vi "decode-from-json.vi"(8 "sensor-options-json":string, 9 "serial-port-json":string, 10 "data-logging-json":string, 11 "filepath-json":string) -> (0 "Sensor Option Recall":T1={"Display Units"="log", "Zero Offset"=2.62, "Sensor Min"=0.0, "Sensor Max"=500.0, "Signal Min"=0.0, "Signal Max"=100.0, "Conversion Factor"=0.0}, 1 "Serial Port Recall":T2={"COM Port (COM10)"="COM10", "baud rate (19200)"=19200, "Simulate Hardware"=FALSE} {"baud rate (19200)" max=115200 step=1200}, 2 "Datalogging Recall":T3={"data-precision"=3, "Include Date"=FALSE, "Include Timestamp"=TRUE, "Include Milliseconds"=FALSE, "sample-rate (Hz)"=4.0, "Logging Active"=TRUE}, 3 "Filepath Recall":T4={"Log Filepath Source"=enum."Application Relative (Auto)", "Log File Path (Manual)"=path "C:/Users/dheard/Documents/0002-labview-projects/ammonia-absorbsion-rig/data", "Log File Folder Name"="data", "log file name"="log", "Include Date in Filename"=TRUE, "Include Time in Filename"=TRUE})   [LabVIEW 2024]
uses:
  csv-file-logging/filepath-selection.ctl
  csv-file-logging/datalogging-options.ctl
  serial-options.ctl
  sensor-options.ctl
  filepath-json-cluster-feck.ctl
  serial-options-json-cluster-feck.ctl
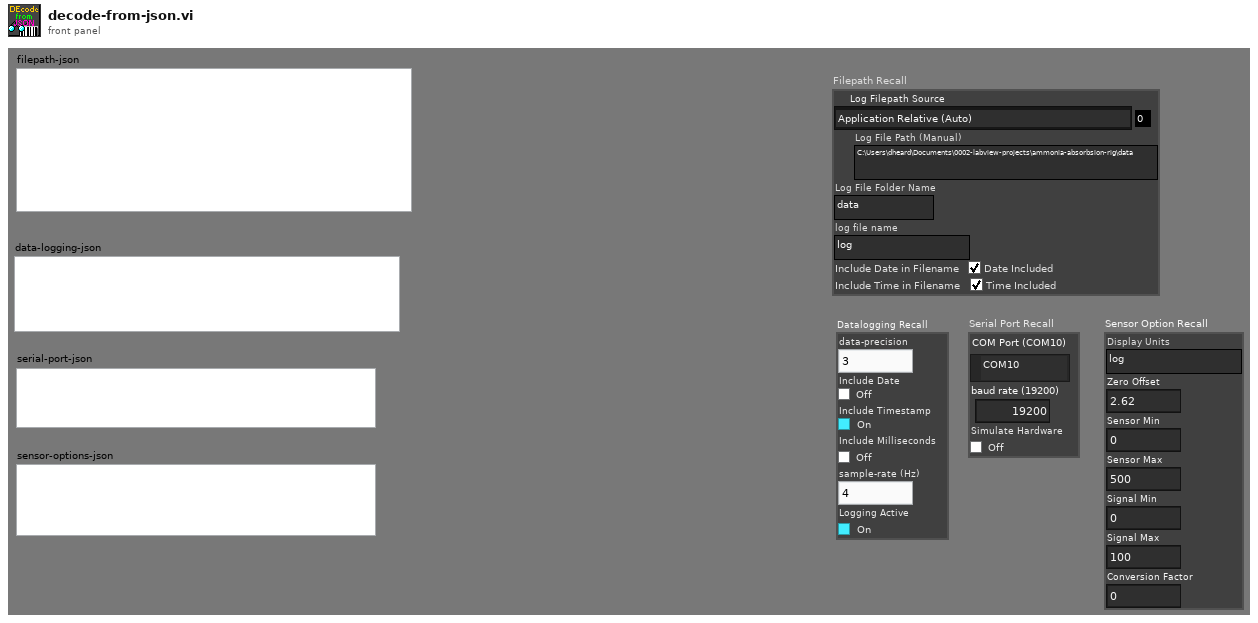
[diagram p1: front panel]
types:
  T1 = typedef "sensor-options.ctl" = cluster{"Display Units":string, "Zero Offset":dbl, "Sensor Min":dbl, "Sensor Max":dbl, "Signal Min":dbl, "Signal Max":dbl, "Conversion Factor":dbl}
  T2 = typedef "serial-options.ctl" = cluster{"COM Port (COM10)":refnum<visa-resource-name>, "baud rate (19200)":u32, "Simulate Hardware":bool}
  T3 = typedef "datalogging-options.ctl" = cluster{"data-precision":i32, "Include Date":bool, "Include Timestamp":bool, "Include Milliseconds":bool, "sample-rate (Hz)":dbl, "Logging Active":bool}
  T4 = typedef "filepath-selection.ctl" = cluster{"Log Filepath Source":enum16{"Application Relative (Auto)", "VI Relative (Auto)", "Complete Path (Manual)"}, "Log File Path (Manual)":path, "Log File Folder Name":string, "log file name":string, "Include Date in Filename":bool, "Include Time in Filename":bool}
  T5 = typedef "serial-options-json-cluster-feck.ctl" = cluster{"unsigned byte array":u8[], "baud rate (19200)":u32, "Simulate Hardware":bool}
  T6 = typedef "filepath-json-cluster-feck.ctl" = cluster{"Log Filepath Source":i32, "Log Filepath byte array":u8[], "Log File Folder Name":string, "log file name":string, "Include Date in Filename":bool, "Include Time in Filename":bool}
  T7 = enum16{"Application Relative (Auto)", "VI Relative (Auto)", "Complete Path (Manual)"}
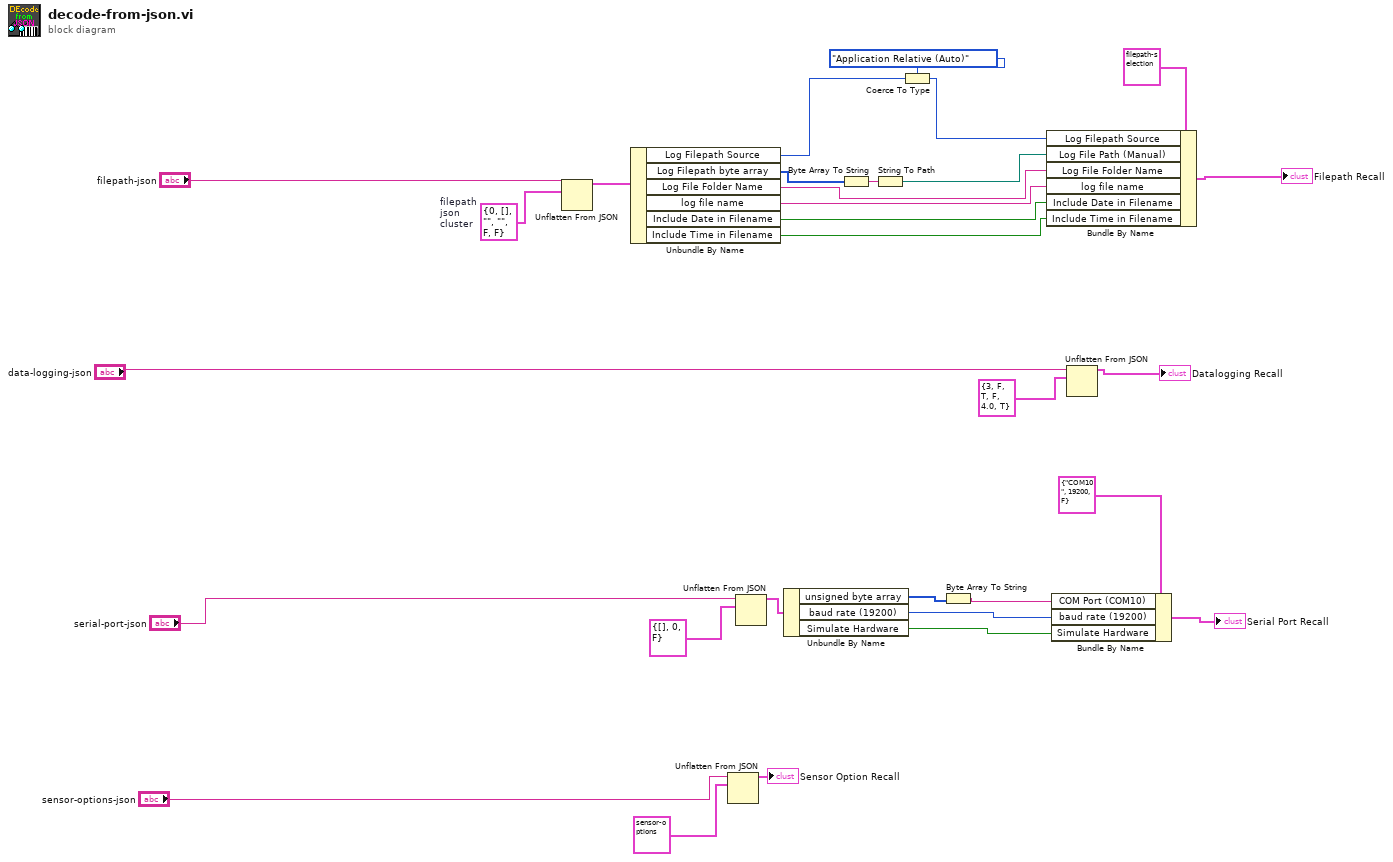
[diagram p0: block diagram]
diagram:
  w16 = T6 {"Log Filepath Source"=0, "Log Filepath byte array"=[], "Log File Folder Name"="", "log file name"="", "Include Date in Filename"=FALSE, "Include Time in Filename"=FALSE}  # filepath json cluster
  n1 = Unflatten From JSON(JSON string="filepath-json", type and defaults=w16) -> (value=w26:T6)  [unwired: 5 in, 1 out]
  n2 = Unbundle By Name(w26) -> ("Log Filepath Source"=w17:i32, "Log Filepath byte array"=w24:u8[], "Log File Folder Name"=w21:string, "log file name"=w20:string, "Include Date in Filename"=w19:bool, "Include Time in Filename"=w18:bool)
  n3 = Unflatten From JSON(JSON string="sensor-options-json", type and defaults=T1 {"Display Units"="units", "Zero Offset"=2.62, "Sensor Min"=0.0, "Sensor Max"=500.0, "Signal Min"=0.0, "Signal Max"=100.0, "Conversion Factor"=0.0} ("Sensor Options")) -> (value=→"Sensor Option Recall":T1)  [unwired: 5 in, 1 out]
  n4 = Unflatten From JSON(JSON string="serial-port-json", type and defaults=T5 {"unsigned byte array"=[], "baud rate (19200)"=0, "Simulate Hardware"=FALSE} ("output cluster")) -> (value=w14:T5)  [unwired: 5 in, 1 out]
  n5 = Unbundle By Name(w14) -> ("unsigned byte array"=w9:u8[], "baud rate (19200)"=w12:u32, "Simulate Hardware"=w11:bool)
  n6 = Byte Array To String(unsigned byte array=w24) -> (string=w23:string)
  n7 = String To Path(string=w23) -> (path=w22:path)
  n8 = Coerce To Type(0:w17, 1:T7."Application Relative (Auto)" ("Log Filepath Source")) -> (2:w28:T7)
  n9 = Byte Array To String(unsigned byte array=w9) -> (string=w8:string)
  n10 = Bundle By Name(cluster=T4 {"Log Filepath Source"=enum."VI Relative (Auto)", "Log File Path (Manual)"=path "C:/Users/dheard/Documents/0002-labview-projects/ammonia-absorbsion-rig/data", "Log File Folder Name"="data", "log file name"="log", "Include Date in Filename"=TRUE, "Include Time in Filename"=TRUE} ("Filepath Selection"), "Log Filepath Source"=w28, "Log File Path (Manual)"=w22, "Log File Folder Name"=w21, "log file name"=w20, "Include Date in Filename"=w19, "Include Time in Filename"=w18) -> (→"Filepath Recall":T4)
  n11 = Bundle By Name(cluster=T2 {"COM Port (COM10)"="COM10", "baud rate (19200)"=19200, "Simulate Hardware"=FALSE} ("Serial Port Options"), "COM Port (COM10)"=w8, "baud rate (19200)"=w12, "Simulate Hardware"=w11) -> (→"Serial Port Recall":T2)
  n12 = Unflatten From JSON(JSON string="data-logging-json", type and defaults=T3 {"data-precision"=3, "Include Date"=FALSE, "Include Timestamp"=TRUE, "Include Milliseconds"=FALSE, "sample-rate (Hz)"=4.0, "Logging Active"=TRUE} ("Datalogging options")) -> (value=→"Datalogging Recall":T3)  [unwired: 5 in, 1 out]
